vi "ToTitleCase.vi"(8 "error in (no error)":errorcluster, 9 "String In":string) -> (0 "error out":errorcluster, 1 "TitleCase Out":string)   [LabVIEW 2024, in "LVarex.lvlib"]
uses:
  C:/Users/bjames/Documents/GitHub/SoundTestX/Support Files/StringCase.dll
  SoundTestX/Support Files/StringCase.dll
  LVarex.lvlib
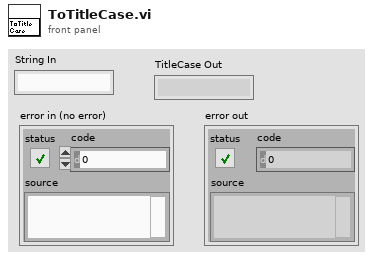
[diagram p1: front panel]
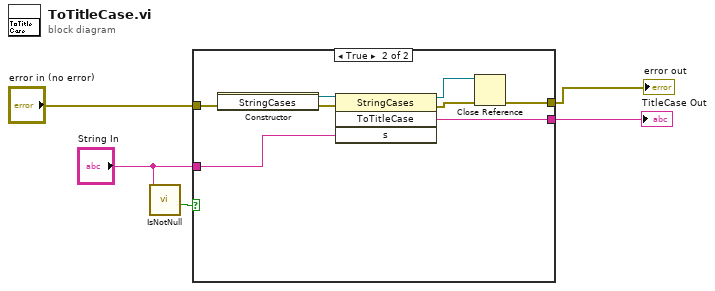
[diagram p0: block diagram]
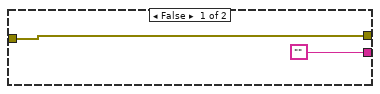
[diagram p2: hidden frame]
diagram:
  n1 = call "IsNotNull.vi"("String In"="String In") -> ("Boolean Out"=w5:bool)  [unwired: 10 in]
  n2 = case shown="True" w5 {
    tunnel: "String In" -> [_ w15]
    tunnel: ["" w14] -> w3
    tunnel: [w6 w11] -> w2
    tunnel: "error in (no error)" -> [w6 w10]
    frame False {
    }
    frame True {
      n3 = constructor class="StringCases"(error in=w10) -> (reference out=w9:refnum<k24>, error out=w8:errorcluster)  [unwired: 2 in, 1 out]
      n4 = invoke class="StringCases" method="ToTitleCase"(reference=w9, error in=w8, "s"=w15) -> (reference out=w13:refnum<k24>, error out=w12:errorcluster, "ToTitleCase"=w14:string)  [unwired: 1 in, 1 out]
      n5 = Close Reference(reference=w13, error in (no error)=w12) -> (error out=w11:errorcluster)
    }
  }
  "TitleCase Out" <- w3
  "error out" <- w2
